vi "Create EventToken.vi"(8 "error in (no error)":errorcluster, 9 "EventRefnum":i32, 10 "EventData Class":refnum<class "EventData.lvclass">) -> (0 "error out":errorcluster, 3 "EventToken out":refnum<class "EventToken.lvclass">)   [LabVIEW 2021, in "EventManagerLibrary.lvlib" / "EventToken.lvclass"]
uses:
  EventToken.lvclass
  EventDataObject/EventData.lvclass
  EventToken.lvclass/EventToken.ctl
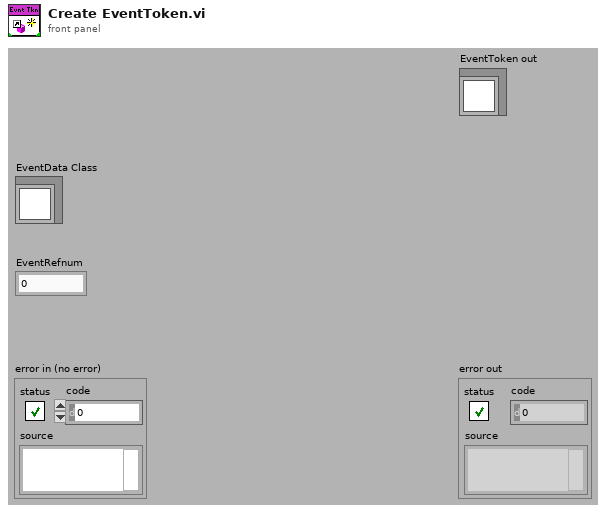
[diagram p1: front panel]
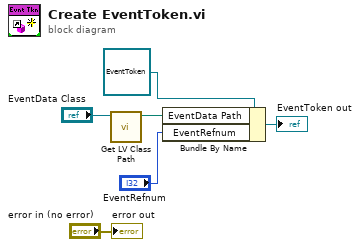
[diagram p0: block diagram]
diagram:
  n1 = call <vilib>:"Get LV Class Path.vi"("object"="EventData Class") -> ("class path"=w1:path)  [unwired: 1 in, 9 out]
  n2 = Bundle By Name(cluster=refnum<class "EventToken.lvclass"> refnum ("EventToken in"), "EventData Path"=w1, "EventRefnum"="EventRefnum") -> (→"EventToken out":refnum<class "EventToken.lvclass">)
  "error out" <- "error in (no error)"
